vi "Set_Flow_Array.vi"(1 "Flow Array":dbl[](array[numeric]), 2 "Index":i32, 3 "Input Sequence":cluster{string, string[], dbl[], dbl}[](array[cluster])) -> (0 "Output Sequence":cluster{string, string[], dbl[], dbl}[](array[cluster]))   [LabVIEW 2011]
doc: "This VI sets the \"Flow Array\" of some event determined by the \"Index\" parameter in the sequence."
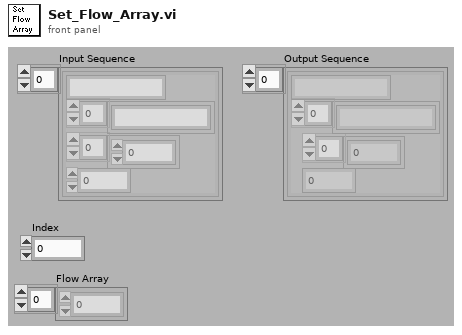
[diagram p1: front panel]
types:
  T1 = cluster{string, string[], "Flow Array":dbl[], dbl}
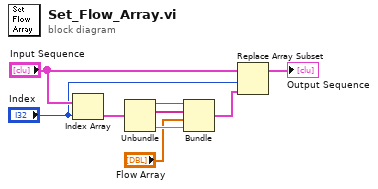
[diagram p0: block diagram]
diagram:
  n1 = Index Array(array="Input Sequence", index="Index") -> (element=w9:cluster{string, string[], dbl[], dbl})
  n2 = Unbundle(w9) -> (w8:string, w7:string[], w6:dbl)  [unwired: 1 out]
  n3 = Bundle(w8, w7, "Flow Array"="Flow Array", w6) -> (w2:T1)  [unwired: 1 out]
  n4 = Replace Array Subset(array="Input Sequence", new element=w2, index="Index") -> (→"Output Sequence":cluster{string, string[], dbl[], dbl}[])
